vi "AFT Linear Prediction (Waveform).vi"(6 "step size":dbl=-1.0, 7 "reset? (F)":bool, 8 "error in (no error)":errorcluster, 10 "signal":waveform(dbl)={"t0"=timestamp(0 s since 1904-01-01), "dt"=0.0, "Y"=[]}, 11 "adaptive filter in":refnum<k20>) -> (0 "error out":errorcluster, 1 "prediction error":waveform(dbl), 3 "adaptive filter out":refnum<k20>, 4 "AR coefficients":dbl[](array[numeric]))   [LabVIEW 2017, in "NI_AdaptiveFilter.lvlib"]
doc: "Performs adaptive linear prediction by estimating the autoregressive (AR) model of an input signal. Wire data to the <B>signal</B> input to determine the polymorphic instance to use or manually select the instance."
uses:
  <vilib>/addons/Adaptive Filters/NI_AdaptiveFilter.lvlib
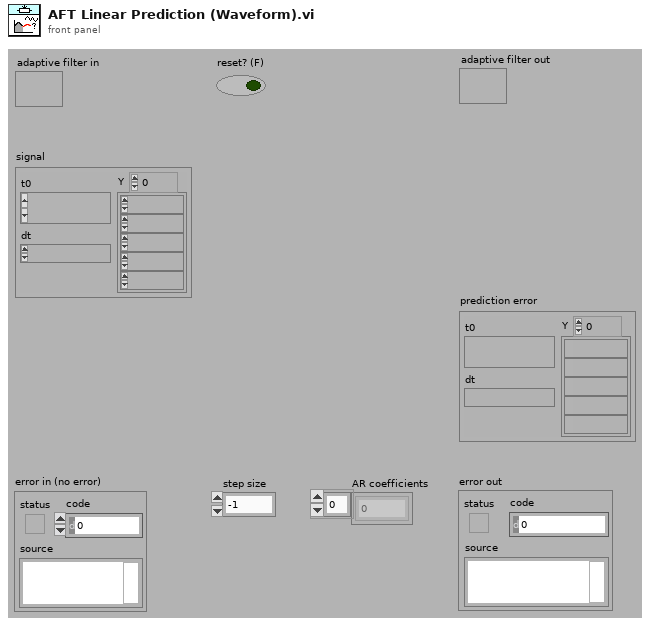
[diagram p1: front panel]
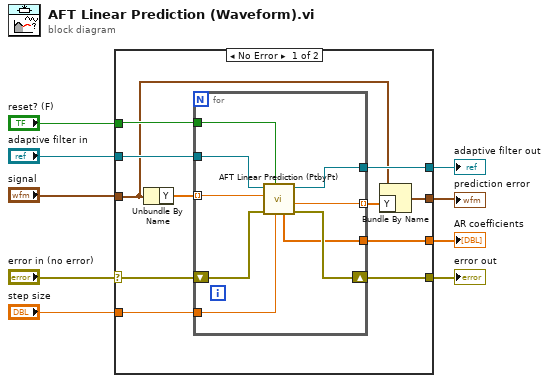
[diagram p0: block diagram]
diagram:
  n1 = case shown="No Error" "error in (no error)" {
    selector: "error in (no error)" -> [w18 w31]
    tunnel: "adaptive filter in" -> [w20 w30]
    tunnel: [w15 w30] -> w8
    tunnel: "signal" -> [w11 _]
    tunnel: [w14 w31] -> w6
    tunnel: "reset? (F)" -> [w19 _]
    tunnel: "step size" -> [w17 _]
    tunnel: [w16 _] -> w3
    tunnel: [w10 _] -> w1
    frame No Error {
      n2 = Unbundle By Name(w11) -> ("Y"=w13:dbl[])
      n3 = for {
        tunnel: w13 -> [w29] mode=indexing
        tunnel: w20 -> [w28]
        tunnel: w19 -> [w27]
        shift-right: [w25] -> w14
        shift-left: w18 -> [w26]
        tunnel: w17 -> [w24]
        tunnel: [w23] -> w16
        tunnel: [w22] -> w15
        tunnel: [w21] -> w12 mode=indexing
        n4 = call <vilib>:"AFT Linear Prediction (PtbyPt).vi"("step size"=w24, "reset? (F)"=w27, "error in (no error)"=w26, "signal"=w29, "adaptive filter in"=w28) -> ("error out"=w25:errorcluster, "prediction error"=w21:dbl, "adaptive filter out"=w22:refnum<k20>, "AR coefficients"=w23:dbl[])  [unwired: 3 out]
      }
      n5 = Bundle By Name(cluster=w11, "Y"=w12) -> (w10:waveform(dbl))
    }
    frame Error {
    }
  }
  "adaptive filter out" <- w8
  "error out" <- w6
  "AR coefficients" <- w3
  "prediction error" <- w1
